vi "VI Tree.vi"   [LabVIEW 2014, in "Stanford Research DG645 - Driver.lvlib"]
doc: "This is the instrument driver for the Stanford Research DG645. The VI Tree displays all the user-callable VIs of the instrument driver in an organized table."
uses:
  Stanford Research DG645 - Driver.lvlib
panel:
  # "(c) 2012 GSI Helmholtzzentrum für Schwerionenforschung GmbH.  ALL RIGHTS RESERVED."
  # "SEE DIAGRAM\nFOR VI TREE."
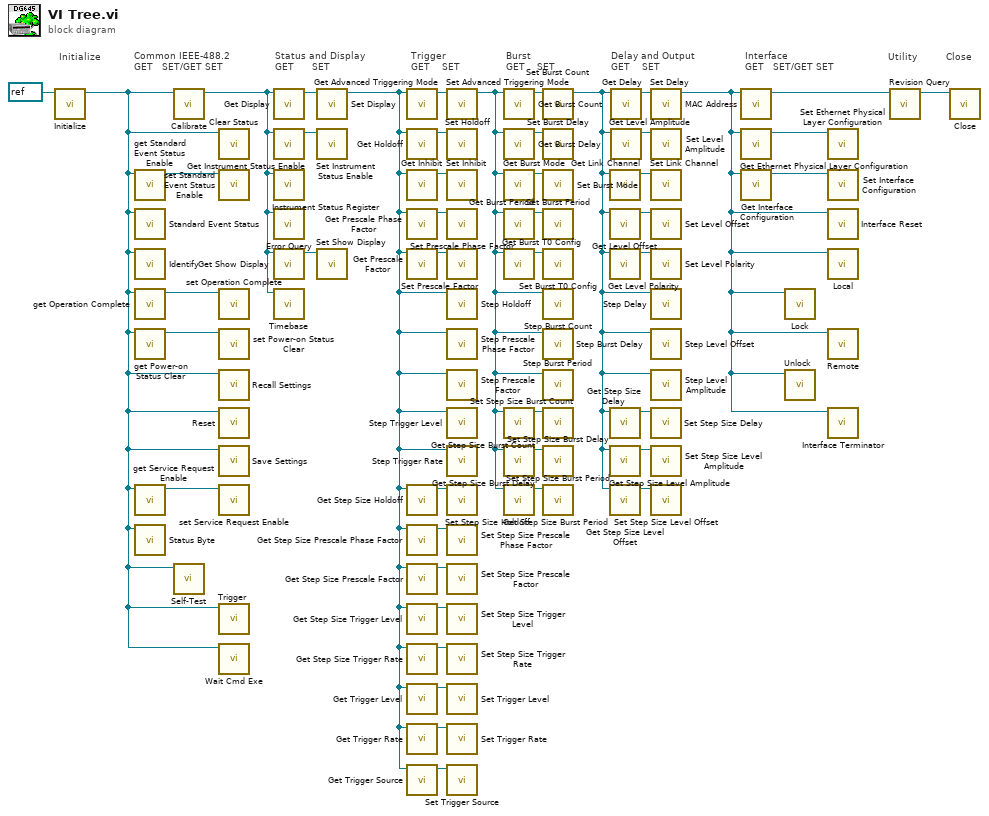
[diagram p0: block diagram]
diagram:
  # "Interface\nGET   SET/GET SET"
  # "Delay and Output\nGET    SET"
  # "Burst\nGET    SET"
  # "Common IEEE-488.2\nGET   SET/GET SET"
  # "Utility"
  # "Trigger\nGET    SET"
  # "Status and Display\nGET      SET"
  # "Close"
  # "Initialize"
  n1 = call "Initialize.vi"("VISA resource name"=refnum<visa-resource-name> refnum) -> ("VISA resource name out"=w42:refnum<visa-resource-name>)  [unwired: 8 in, 2 out]
  n2 = call "get Standard Event Status Enable.vi"("VISA resource name"=w42) -> ("VISA resource name out"=w44:refnum<visa-resource-name>)  [unwired: 7 in, 3 out]
  n3 = call "Standard Event Status.vi"("VISA resource name"=w42) -> ()  [unwired: 6 in, 5 out]
  n4 = call "Identify.vi"("VISA resource name"=w42) -> ()  [unwired: 3 in, 8 out]
  n5 = call "get Operation Complete.vi"("VISA resource name"=w42) -> ("VISA resource name out"=w45:refnum<visa-resource-name>)  [unwired: 6 in, 4 out]
  n6 = call "get Power-on Status Clear.vi"("VISA resource name"=w42) -> ("VISA resource name out"=w43:refnum<visa-resource-name>)  [unwired: 7 in, 3 out]
  n7 = call "get Service Request Enable.vi"("VISA resource name"=w42) -> ("VISA resource name out"=w41:refnum<visa-resource-name>)  [unwired: 7 in, 3 out]
  n8 = call "Status Byte.vi"("VISA resource name"=w42) -> ()  [unwired: 6 in, 5 out]
  n9 = call "Calibrate.vi"("VISA resource name"=w42) -> ("VISA resource name out"=w37:refnum<visa-resource-name>)  [unwired: 6 in, 4 out]
  n10 = call "Self-Test.vi"("VISA resource name"=w42) -> ()  [unwired: 6 in, 5 out]
  n11 = call "Clear Status.vi"("VISA resource name"=w42) -> ()  [unwired: 8 in, 3 out]
  n12 = call "set Standard Event Status Enable.vi"("VISA resource name"=w44) -> ()  [unwired: 8 in, 3 out]
  n13 = call "set Operation Complete.vi"("VISA resource name"=w45) -> ()  [unwired: 8 in, 3 out]
  n14 = call "set Power-on Status Clear.vi"("VISA resource name"=w43) -> ()  [unwired: 8 in, 3 out]
  n15 = call "Recall Settings.vi"("VISA resource name"=w42) -> ()  [unwired: 8 in, 3 out]
  n16 = call "Reset.vi"("VISA resource name"=w42) -> ()  [unwired: 8 in, 3 out]
  n17 = call "Save Settings.vi"("VISA resource name"=w42) -> ()  [unwired: 8 in, 3 out]
  n18 = call "set Service Request Enable.vi"("VISA resource name"=w41) -> ()  [unwired: 8 in, 3 out]
  n19 = call "Trigger.vi"("VISA resource name"=w42) -> ()  [unwired: 8 in, 3 out]
  n20 = call "Wait Cmd Exe.vi"("VISA resource name"=w42) -> ()  [unwired: 8 in, 3 out]
  n21 = call "Get Display.vi"("VISA resource name"=w37) -> ("VISA resource name out"=w38:refnum<visa-resource-name>)  [unwired: 6 in, 4 out]
  n22 = call "Get Instrument Status Enable.vi"("VISA resource name"=w37) -> ("VISA resource name out"=w39:refnum<visa-resource-name>)  [unwired: 7 in, 3 out]
  n23 = call "Instrument Status Register.vi"("VISA resource name"=w37) -> ()  [unwired: 6 in, 5 out]
  n24 = call "Error Query.vi"("VISA resource name"=w37) -> ()  [unwired: 8 in, 3 out]
  n25 = call "Get Show Display.vi"("VISA resource name"=w37) -> ("VISA resource name out"=w40:refnum<visa-resource-name>)  [unwired: 7 in, 3 out]
  n26 = call "Timebase.vi"("VISA resource name"=w37) -> ()  [unwired: 7 in, 4 out]
  n27 = call "Set Display.vi"("VISA resource name"=w38) -> ("VISA resource name out"=w6:refnum<visa-resource-name>)  [unwired: 8 in, 2 out]
  n28 = call "Set Instrument Status Enable.vi"("VISA resource name"=w39) -> ()  [unwired: 8 in, 3 out]
  n29 = call "Set Show Display.vi"("VISA resource name"=w40) -> ()  [unwired: 8 in, 3 out]
  n30 = call "Get Advanced Triggering Mode.vi"("VISA resource name"=w6) -> ("VISA resource name out"=w26:refnum<visa-resource-name>)  [unwired: 7 in, 3 out]
  n31 = call "Get Holdoff.vi"("VISA resource name"=w6) -> ("VISA resource name out"=w25:refnum<visa-resource-name>)  [unwired: 7 in, 3 out]
  n32 = call "Get Inhibit.vi"("VISA resource name"=w6) -> ("VISA resource name out"=w24:refnum<visa-resource-name>)  [unwired: 7 in, 3 out]
  n33 = call "Get Prescale Phase Factor.vi"("VISA resource name"=w6) -> ("VISA resource name out"=w23:refnum<visa-resource-name>)  [unwired: 7 in, 3 out]
  n34 = call "Get Prescale Factor.vi"("VISA resource name"=w6) -> ("VISA resource name out"=w22:refnum<visa-resource-name>)  [unwired: 7 in, 3 out]
  n35 = call "Get Step Size Holdoff.vi"("VISA resource name"=w6) -> ("VISA resource name out"=w5:refnum<visa-resource-name>)  [unwired: 7 in, 3 out]
  n36 = call "Get Step Size Prescale Phase Factor.vi"("VISA resource name"=w6) -> ("VISA resource name out"=w4:refnum<visa-resource-name>)  [unwired: 7 in, 3 out]
  n37 = call "Get Step Size Prescale Factor.vi"("VISA resource name"=w6) -> ("VISA resource name out"=w3:refnum<visa-resource-name>)  [unwired: 7 in, 3 out]
  n38 = call "Get Step Size Trigger Level.vi"("VISA resource name"=w6) -> ("VISA resource name out"=w2:refnum<visa-resource-name>)  [unwired: 7 in, 3 out]
  n39 = call "Get Step Size Trigger Rate.vi"("VISA resource name"=w6) -> ("VISA resource name out"=w1:refnum<visa-resource-name>)  [unwired: 7 in, 3 out]
  n40 = call "Get Trigger Level.vi"("VISA resource name"=w6) -> ("VISA resource name out"=w21:refnum<visa-resource-name>)  [unwired: 7 in, 3 out]
  n41 = call "Get Trigger Rate.vi"("VISA resource name"=w6) -> ("VISA resource name out"=w20:refnum<visa-resource-name>)  [unwired: 7 in, 3 out]
  n42 = call "Get Trigger Source.vi"("VISA resource name"=w6) -> ("VISA resource name out"=w19:refnum<visa-resource-name>)  [unwired: 7 in, 3 out]
  n43 = call "Set Advanced Triggering Mode.vi"("VISA resource name"=w26) -> ("VISA resource name out"=w14:refnum<visa-resource-name>)  [unwired: 8 in, 2 out]
  n44 = call "Set Holdoff.vi"("VISA resource name"=w25) -> ()  [unwired: 8 in, 3 out]
  n45 = call "Set Inhibit.vi"("VISA resource name"=w24) -> ()  [unwired: 8 in, 3 out]
  n46 = call "Set Prescale Phase Factor.vi"("VISA resource name"=w23) -> ()  [unwired: 8 in, 3 out]
  n47 = call "Set Prescale Factor.vi"("VISA resource name"=w22) -> ()  [unwired: 8 in, 3 out]
  n48 = call "Step Holdoff.vi"("VISA resource name"=w6) -> ()  [unwired: 8 in, 3 out]
  n49 = call "Step Prescale Phase Factor.vi"("VISA resource name"=w6) -> ()  [unwired: 8 in, 3 out]
  n50 = call "Step Prescale Factor.vi"("VISA resource name"=w6) -> ()  [unwired: 8 in, 3 out]
  n51 = call "Step Trigger Level.vi"("VISA resource name"=w6) -> ()  [unwired: 8 in, 3 out]
  n52 = call "Step Trigger Rate.vi"("VISA resource name"=w6) -> ()  [unwired: 8 in, 3 out]
  n53 = call "Set Step Size Holdoff.vi"("VISA resource name"=w5) -> ()  [unwired: 8 in, 3 out]
  n54 = call "Set Step Size Prescale Phase Factor.vi"("VISA resource name"=w4) -> ()  [unwired: 8 in, 3 out]
  n55 = call "Set Step Size Prescale Factor.vi"("VISA resource name"=w3) -> ()  [unwired: 8 in, 3 out]
  n56 = call "Set Step Size Trigger Level.vi"("VISA resource name"=w2) -> ()  [unwired: 8 in, 3 out]
  n57 = call "Set Step Size Trigger Rate.vi"("VISA resource name"=w1) -> ()  [unwired: 8 in, 3 out]
  n58 = call "Set Trigger Level.vi"("VISA resource name"=w21) -> ()  [unwired: 8 in, 3 out]
  n59 = call "Set Trigger Rate.vi"("VISA resource name"=w20) -> ()  [unwired: 8 in, 3 out]
  n60 = call "Set Trigger Source.vi"("VISA resource name"=w19) -> ()  [unwired: 8 in, 3 out]
  n61 = call "Get Burst Count.vi"("VISA resource name"=w14) -> ("VISA resource name out"=w31:refnum<visa-resource-name>)  [unwired: 7 in, 3 out]
  n62 = call "Get Burst Delay.vi"("VISA resource name"=w14) -> ("VISA resource name out"=w30:refnum<visa-resource-name>)  [unwired: 7 in, 3 out]
  n63 = call "Get Burst Mode.vi"("VISA resource name"=w14) -> ("VISA resource name out"=w29:refnum<visa-resource-name>)  [unwired: 7 in, 3 out]
  n64 = call "Get Burst Period.vi"("VISA resource name"=w14) -> ("VISA resource name out"=w28:refnum<visa-resource-name>)  [unwired: 7 in, 3 out]
  n65 = call "Get Burst T0 Config.vi"("VISA resource name"=w14) -> ("VISA resource name out"=w27:refnum<visa-resource-name>)  [unwired: 7 in, 3 out]
  n66 = call "Get Step Size Burst Count.vi"("VISA resource name"=w14) -> ("VISA resource name out"=w13:refnum<visa-resource-name>)  [unwired: 7 in, 3 out]
  n67 = call "Get Step Size Burst Delay.vi"("VISA resource name"=w14) -> ("VISA resource name out"=w12:refnum<visa-resource-name>)  [unwired: 7 in, 3 out]
  n68 = call "Get Step Size Burst Period.vi"("VISA resource name"=w14) -> ("VISA resource name out"=w11:refnum<visa-resource-name>)  [unwired: 7 in, 3 out]
  n69 = call "Set Burst Count.vi"("VISA resource name"=w31) -> ("VISA resource name out"=w10:refnum<visa-resource-name>)  [unwired: 8 in, 2 out]
  n70 = call "Set Burst Delay.vi"("VISA resource name"=w30) -> ()  [unwired: 8 in, 3 out]
  n71 = call "Set Burst Mode.vi"("VISA resource name"=w29) -> ()  [unwired: 8 in, 3 out]
  n72 = call "Set Burst Period.vi"("VISA resource name"=w28) -> ()  [unwired: 8 in, 3 out]
  n73 = call "Set Burst T0 Config.vi"("VISA resource name"=w27) -> ()  [unwired: 8 in, 3 out]
  n74 = call "Step Burst Count.vi"("VISA resource name"=w14) -> ()  [unwired: 8 in, 3 out]
  n75 = call "Step Burst Delay.vi"("VISA resource name"=w14) -> ()  [unwired: 8 in, 3 out]
  n76 = call "Step Burst Period.vi"("VISA resource name"=w14) -> ()  [unwired: 8 in, 3 out]
  n77 = call "Set Step Size Burst Count.vi"("VISA resource name"=w13) -> ()  [unwired: 8 in, 3 out]
  n78 = call "Set Step Size Burst Delay.vi"("VISA resource name"=w12) -> ()  [unwired: 8 in, 3 out]
  n79 = call "Set Step Size Burst Period.vi"("VISA resource name"=w11) -> ()  [unwired: 8 in, 3 out]
  n80 = call "Get Link Channel.vi"("VISA resource name"=w10) -> ("VISA resource name out"=w34:refnum<visa-resource-name>)  [unwired: 7 in, 3 out]
  n81 = call "Get Level Offset.vi"("VISA resource name"=w10) -> ("VISA resource name out"=w33:refnum<visa-resource-name>)  [unwired: 7 in, 3 out]
  n82 = call "Get Level Polarity.vi"("VISA resource name"=w10) -> ("VISA resource name out"=w32:refnum<visa-resource-name>)  [unwired: 7 in, 3 out]
  n83 = call "Get Step Size Delay.vi"("VISA resource name"=w10) -> ("VISA resource name out"=w9:refnum<visa-resource-name>)  [unwired: 7 in, 3 out]
  n84 = call "Get Step Size Level Amplitude.vi"("VISA resource name"=w10) -> ("VISA resource name out"=w8:refnum<visa-resource-name>)  [unwired: 7 in, 3 out]
  n85 = call "Get Step Size Level Offset.vi"("VISA resource name"=w10) -> ("VISA resource name out"=w7:refnum<visa-resource-name>)  [unwired: 7 in, 3 out]
  n86 = call "Get Delay.vi"("VISA resource name"=w10) -> ("VISA resource name out"=w36:refnum<visa-resource-name>)  [unwired: 6 in, 4 out]
  n87 = call "Get Level Amplitude.vi"("VISA resource name"=w10) -> ("VISA resource name out"=w35:refnum<visa-resource-name>)  [unwired: 7 in, 3 out]
  n88 = call "Set Delay.vi"("VISA resource name"=w36) -> ("VISA resource name out"=w15:refnum<visa-resource-name>)  [unwired: 8 in, 2 out]
  n89 = call "Set Level Amplitude.vi"("VISA resource name"=w35) -> ()  [unwired: 8 in, 3 out]
  n90 = call "Set Link Channel.vi"("VISA resource name"=w34) -> ()  [unwired: 8 in, 3 out]
  n91 = call "Set Level Offset.vi"("VISA resource name"=w33) -> ()  [unwired: 8 in, 3 out]
  n92 = call "Set Level Polarity.vi"("VISA resource name"=w32) -> ()  [unwired: 8 in, 3 out]
  n93 = call "Step Delay.vi"("VISA resource name"=w10) -> ()  [unwired: 8 in, 3 out]
  n94 = call "Step Level Offset.vi"("VISA resource name"=w10) -> ()  [unwired: 8 in, 3 out]
  n95 = call "Step Level Amplitude.vi"("VISA resource name"=w10) -> ()  [unwired: 8 in, 3 out]
  n96 = call "Set Step Size Delay.vi"("VISA resource name"=w9) -> ()  [unwired: 8 in, 3 out]
  n97 = call "Set Step Size Level Amplitude.vi"("VISA resource name"=w8) -> ()  [unwired: 8 in, 3 out]
  n98 = call "Set Step Size Level Offset.vi"("VISA resource name"=w7) -> ()  [unwired: 8 in, 3 out]
  n99 = call "MAC Address.vi"("VISA resource name"=w15) -> ("VISA resource name out"=w18:refnum<visa-resource-name>)  [unwired: 7 in, 3 out]
  n100 = call "Get Ethernet Physical Layer Configuration.vi"("VISA resource name"=w15) -> ("VISA resource name out"=w17:refnum<visa-resource-name>)  [unwired: 7 in, 3 out]
  n101 = call "Get Interface Configuration.vi"("VISA resource name"=w15) -> ("VISA resource name out"=w16:refnum<visa-resource-name>)  [unwired: 7 in, 3 out]
  n102 = call "Lock.vi"("VISA resource name"=w15) -> ()  [unwired: 7 in, 4 out]
  n103 = call "Unlock.vi"("VISA resource name"=w15) -> ()  [unwired: 7 in, 4 out]
  n104 = call "Set Ethernet Physical Layer Configuration.vi"("VISA resource name"=w17) -> ()  [unwired: 8 in, 3 out]
  n105 = call "Set Interface Configuration.vi"("VISA resource name"=w16) -> ()  [unwired: 8 in, 3 out]
  n106 = call "Interface Reset.vi"("VISA resource name"=w15) -> ()  [unwired: 8 in, 3 out]
  n107 = call "Local.vi"("VISA resource name"=w15) -> ()  [unwired: 8 in, 3 out]
  n108 = call "Remote.vi"("VISA resource name"=w15) -> ()  [unwired: 8 in, 3 out]
  n109 = call "Interface Terminator.vi"("VISA resource name"=w15) -> ()  [unwired: 8 in, 3 out]
  n110 = call "Revision Query.vi"("VISA resource name"=w18) -> ("VISA resource name out"=w46:refnum<visa-resource-name>)  [unwired: 6 in, 4 out]
  n111 = call "Close.vi"("VISA resource name"=w46) -> ()  [unwired: 9 in, 2 out]
